vi "Append Buffer to File in the USB.vi"(0 "VISA resource name":refnum<visa-resource-name>, 1 "Enable Time Format (F:Disable)":bool, 2 "Enable Start & End (F:Disable)":bool, 5 "Buffer Name (defbuffer1)":string="defbuffer1", 7 "File Name":string, 9 "Time Format":u16(ring) items=["Format", "Relative", "Raw", "Stamp"], 11 "error in (no error)":errorcluster, 12 "Start":i32, 13 "End":i32) -> (4 "VISA resource name out":refnum<visa-resource-name>, 15 "error out":errorcluster)   [LabVIEW 2015, in "Keithley 2450.lvlib"]
doc: "This VI appends data from the reading buffer to a file on the USB flash drive."
uses:
  <instrlib>/Keithley 2450/Keithley 2450.lvlib
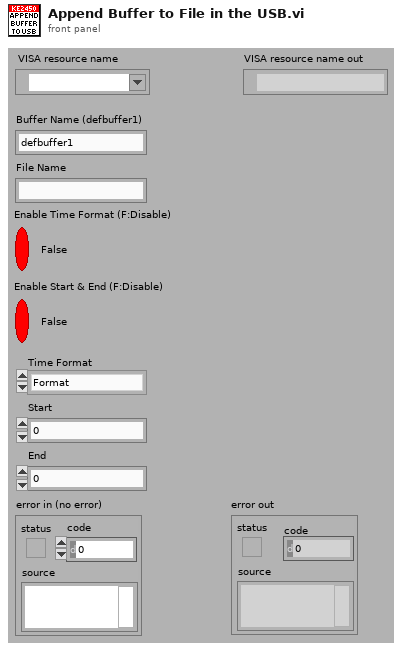
[diagram p1: front panel]
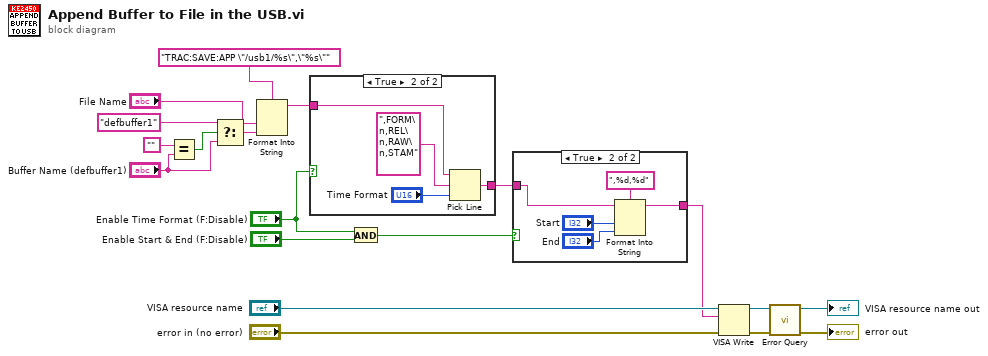
[diagram p0: block diagram]
diagram:
  n1 = Equal?(x="", y="Buffer Name (defbuffer1)") -> (x = y?=w11:bool)
  n2 = Select(t="defbuffer1", s=w11, f="Buffer Name (defbuffer1)") -> (s? t:f=w7:string)
  n3 = Format Into String(format string="TRAC:SAVE:APP \"/usb1/%s\",\"%s\"" ("Read Measurement"), "File Name", w7) -> (resulting string=w3:string)  [unwired: 2 in, 1 out]
  n4 = case shown="True" "Enable Time Format (F:Disable)" {
    tunnel: [w20 w22] -> w2
    tunnel: w3 -> [w20 w21]
    frame False {
    }
    frame True {
      n5 = Pick Line(string ("")=w21, multi-line string=",FORM\n,REL\n,RAW\n,STAM", line index="Time Format") -> (output string=w22:string)
    }
  }
  n6 = And(x="Enable Time Format (F:Disable)", y="Enable Start & End (F:Disable)") -> (x .and. y?=w5:bool)
  n7 = case shown="True" w5 {
    tunnel: w2 -> [w25 w27]
    tunnel: [w25 w26] -> w1
    frame False {
    }
    frame True {
      n8 = Format Into String(format string=",%d,%d", initial string=w27, "Start", "End") -> (resulting string=w26:string)  [unwired: 1 in, 1 out]
    }
  }
  n9 = VISA Write(VISA resource name="VISA resource name", write buffer=w1, error in (no error)="error in (no error)") -> (VISA resource name out=w15:refnum<visa-resource-name>, error out=w14:errorcluster)  [unwired: 1 out]
  n10 = call <instrlib>:"Error Query.vi"("error in (no error)"=w14, "VISA resource name"=w15) -> ("error out"=→"error out":errorcluster, "VISA resource name out"=→"VISA resource name out":refnum<visa-resource-name>)  [unwired: 8 out]
